vi "CamHandle.vi"() -> ()   [LabVIEW 2015]
panel:
  out "Camera Opened":bool
  in  "Y dimension":u32
  in  "X dimension":u32
  in  "Cam Handle":u32
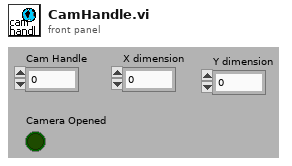
[diagram p1: front panel]
diagram:
